vi "pixelfly_close.vi"(2 "error in (no error)":errorcluster, 3 "Acquitsition Settings":T1) -> (0 "error out":errorcluster)   [LabVIEW 2016]
doc: "This VI stops the PixelFly camera, frees up memory (camera and buffer), and releases the camera board from computer control."
uses:
  Controls/PixelFly/Acquisition Settings.ctl
  <vilib>/Utility/error.llb/DialogType.ctl
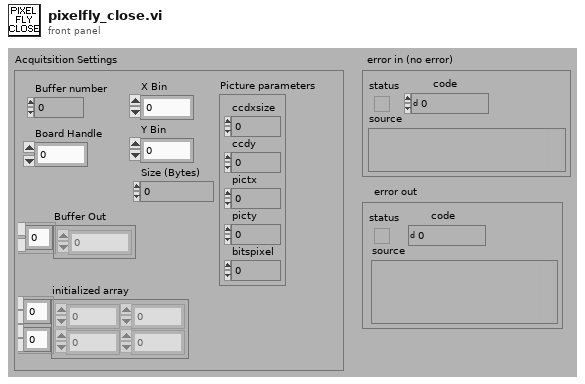
[diagram p1: front panel]
types:
  T1 = typedef "Acquisition Settings.ctl" = cluster{"Buffer number":i32, "Size (Bytes)":i32, "initialized array":u16[][], "X Bin":i32, "Y Bin":i32, "Board Handle":u32, "Picture parameters":cluster{"ccdxsize":i32, "ccdy":i32, "pictx":i32, "picty":i32, "bitspixel":i32}, "Buffer Out":u16[]}
  T2 = typedef "DialogType.ctl" = u16
  T3 = cluster{"Write":bool, "Write done":bool, "Queued":bool, "Cancelled":bool, "Select":bool, "Select done":bool, "Burst":bool, "Size":bool, "Event":bool, "Timeout":bool, "Open":i32, "Map":i32, "Exposure":i32[], "Offset":i32[], "Size":i32[], "Transfer":i32[], "Total Size":i32}
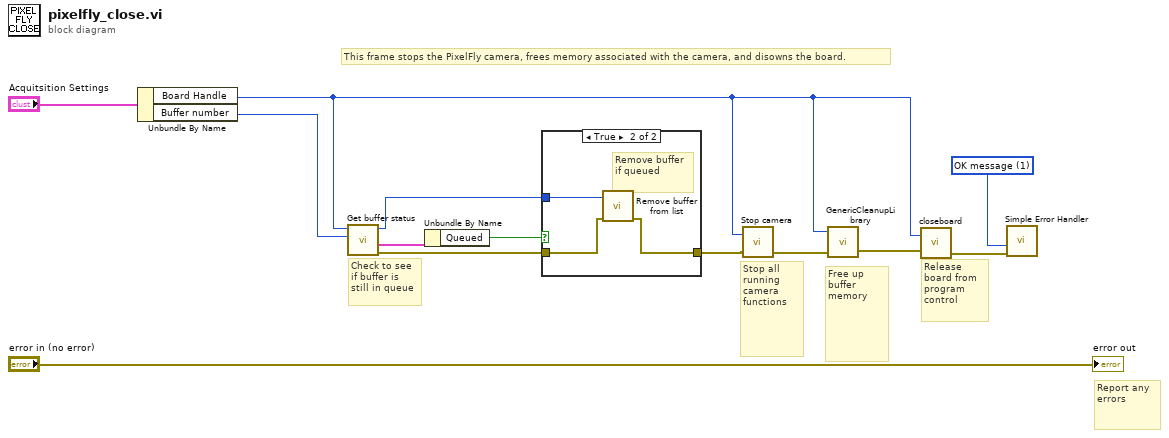
[diagram p0: block diagram]
diagram:
  w1 = T2 1 items=["no dialog", "OK message", "continue or stop message", "OK message + warnings", "continue/stop + warnings"] ("type of dialog (OK msg:1)")
  # "This frame stops the PixelFly camera, frees memory associated with the camera, and disowns the board."
  # "Check to see if buffer is still in queue"
  # "Release board from program control"
  # "Free up buffer memory"
  # "Stop all running camera functions"
  # "Report any errors"
  n1 = Unbundle By Name("Acquitsition Settings") -> ("Board Handle"=w4:u32, "Buffer number"=w7:i32)
  n2 = call "Get buffer status.vi"("Buffer request"=w7, "Handle in"=w4) -> ("error out"=w11:errorcluster, "Buffer status"=w12:T3, "Handle out"=w8:u32)  [unwired: 2 in, 1 out]
  n3 = Unbundle By Name(w12) -> ("Queued"=w10:bool)
  n4 = case shown="True" w10 {
    tunnel: w11 -> [w14 w17]
    tunnel: [w14 w16] -> w9
    tunnel: w8 -> [_ w15]
    frame False {
      # "Successfull write has removed buffer from queue"
    }
    frame True {
      # "Remove buffer if queued"
      n5 = call "Remove buffer from list.vi"("error in (no error)"=w17, "Handle in"=w15) -> ("error out"=w16:errorcluster)  [unwired: 4 in, 1 out]
    }
  }
  n6 = call "Stop camera.vi"("Handle in"=w4, "error in (no error)"=w9) -> ("error out"=w6:errorcluster)  [unwired: 2 out]
  n7 = call "GenericCleanupLibrary.vi"("error in (no error)"=w6, "hIn"=w4) -> ("error out"=w5:errorcluster)  [unwired: 2 in]
  n8 = call "closeboard.vi"("Handle in"=w4, "error in (no error)"=w5) -> ("error out"=w2:errorcluster)  [unwired: 2 out]
  n9 = call <vilib>:"Simple Error Handler.vi"("type of dialog (OK msg:1)"=w1, "error in (no error)"=w2) -> ()  [unwired: 3 in, 5 out]
  "error out" <- "error in (no error)"
